vi "Get FPGA Bitfile.vi"(8 "error in":errorcluster, 10 "Target.Type":T1, 11 "VS Engine in":refnum<class "VS Engine.lvclass">) -> (0 "error out":errorcluster, 2 "Path":path, 3 "VS Engine out":refnum<class "VS Engine.lvclass">)   [LabVIEW 2024, in "VS Engine Abstraction.lvlib" / "VS Engine.lvclass"]
uses:
  VS Engine.lvclass
  VS Engine.lvclass/VS Engine.ctl
  <vilib>/NI VeriStand/Custom Device API/Custom Device API.lvlib
  Addon Shared/SubVIs/Constants.vi
  Addon Shared/FPGA Addon Shared.lvlib
  <vilib>/NI VeriStand/Custom Device API/Get Item Property (Dependent File).vi
  <vilib>/NI VeriStand/Custom Device API/Custom Device Target Type.ctl
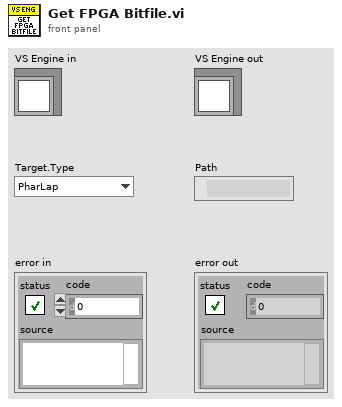
[diagram p1: front panel]
types:
  T1 = typedef "Custom Device API.lvlib/Custom Device Target Type.ctl" = enum16{"PharLap", "VxWorks", "Windows", "Linux_32_ARM", "Linux_x64"}
  T2 = typedef "Custom Device API.lvlib/Custom Device Item Ref.ctl" = u64
  T3 = typedef "Custom Device API.lvlib/Dependent File Optional Info.ctl" = cluster{"Version":string, "RTDestination":path, "ForceDownload":bool, "SupportedTarget":string, "MD5":string}
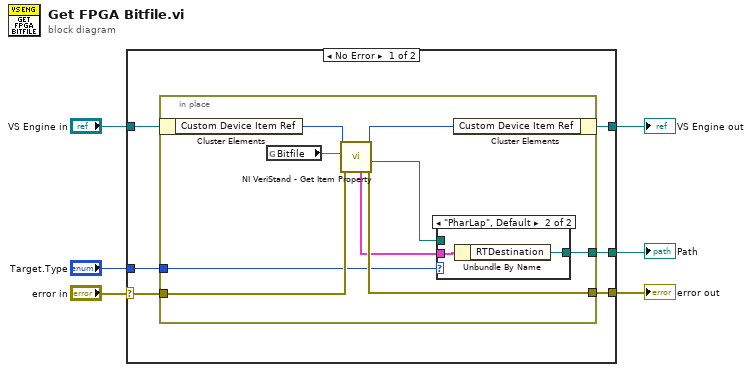
[diagram p0: block diagram]
diagram:
  n1 = case shown="No Error" "error in" {
    selector: "error in" -> [w12 w26]
    tunnel: [w11 w26] -> w5
    tunnel: [w10 _] -> w4
    tunnel: "VS Engine in" -> [w9 w25]
    tunnel: [w8 w25] -> w2
    tunnel: "Target.Type" -> [w7 _]
    frame No Error {
      n2 = in-place {
        in-place-border: w12 -> [w21]
        in-place-border: [w20] -> w11
        in-place-border: [w16] -> w10
        in-place-border: w7 -> [w13]
        n3 = in-place-cluster #1(w9) -> ("Custom Device Item Ref"=w15:T2)
        n4 = global read "Constants.vi" "Bitfile"() -> (w19:string)
        n5 = call-poly <vilib>:"NI VeriStand - Get Item Property.vi"("error in (no error)"=w21, "Property Name"=w19, "Item Ref in"=w15) -> ("error out"=w20:errorcluster, "Path"=w18:path, "Item Ref out"=w14:T2, "OptionalInfo"=w17:T3)  [unwired: 4 in, 1 out]
        n6 = case shown="\"PharLap\", Default" w13 {
          tunnel: w17 -> [_ w24]
          tunnel: [w22 w23] -> w16
          tunnel: w18 -> [w22 _]
          frame "Windows" {
          }
          frame "PharLap", Default {
            n7 = Unbundle By Name(w24) -> ("RTDestination"=w23:path)
          }
        }
        n8 = in-place-cluster #1("Custom Device Item Ref"=w14) -> (w8:refnum<class "VS Engine.lvclass">)
      }
    }
    frame Error {
    }
  }
  "VS Engine out" <- w2
  "error out" <- w5
  "Path" <- w4
